vi "ISMBUS_DecodeModuleBaudRate.vi"(8 "Fehler (Eingang - kein Fehler)":errorcluster, 11 "ModuleBaudRate in":i32) -> (0 "error (Ausgang)":errorcluster caption="Fehler  (Ausgang)", 3 "ModuleBaudRate in 2":i32)   [LabVIEW 2016]
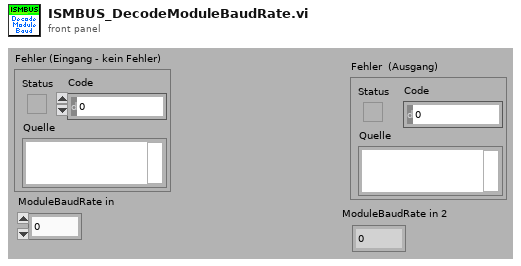
[diagram p1: front panel]
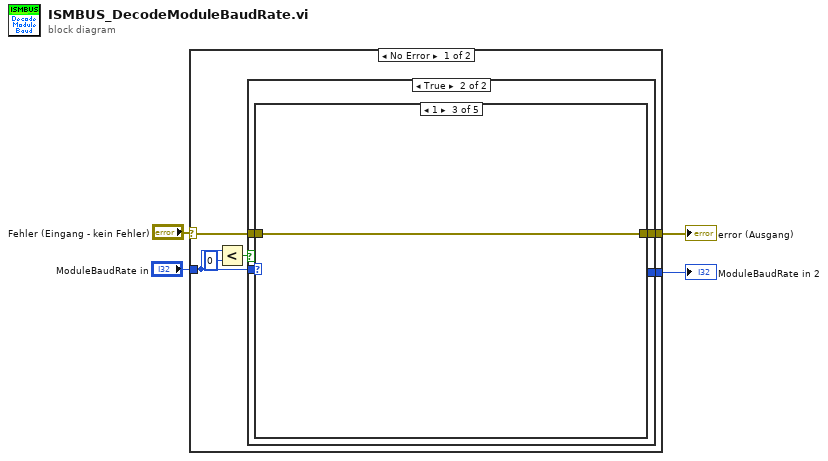
[diagram p0: block diagram]
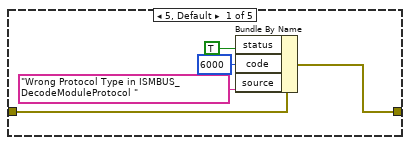
[diagram p3: hidden frame]
diagram:
  n1 = case shown="No Error" "Fehler (Eingang - kein Fehler)" {
    selector: "Fehler (Eingang - kein Fehler)" -> [w10 w25]
    tunnel: "ModuleBaudRate in" -> [w8 _]
    tunnel: [w9 w25] -> w3
    tunnel: [w5 _] -> w1
    frame No Error {
      n2 = Less?(x=w8, y=0) -> (x < y?=w6:bool)
      n3 = case shown="True" w6 {
        tunnel: w8 -> [w12 w15]
        tunnel: w10 -> [w11 w14]
        tunnel: [w11 w13] -> w9
        tunnel: [w12 _] -> w5
        frame False {
        }
        frame True {
          n4 = case shown="1" w15 {
            tunnel: w14 -> [w19 w21 w22 w23 w24]
            tunnel: [w20 w21 w22 w23 w24] -> w13
            frame 5, Default {
              n5 = Bundle By Name(cluster=w19, "status"=TRUE, "code"=6000, "source"="Wrong Protocol Type in ISMBUS_DecodeModuleProtocol ") -> (w20:errorcluster)
            }
            frame 0 {
            }
            frame 1 {
            }
            frame 2 {
            }
            frame 3 {
            }
          }
        }
      }
    }
    frame Error {
    }
  }
  "error (Ausgang)" <- w3
  "ModuleBaudRate in 2" <- w1
